vi "NXT_MIDBRAIN REVERSE.vi"(2 "_sensorData":T2={"_irData"={"_irDistance"=0, "_irHeading"=0, "_irTimestamp"=0}, "_batteryVoltage"=0, "_NXTButtonStates"=[FALSE, FALSE, FALSE]}, 3 "Behavior #":i32, 4 "Previous Motor Position":T1={"_rudderCommand"=7, "_propCommand"=7, "_irServoCommand"=7}, 5 "Behavior Weights":T4=[0, 0, 0, 0, 0, 0]) -> (0 "Rudder Command":i32, 1 "Behavior Output":T5)   [LabVIEW 2012]
uses:
  behaviorOutput_t.ctl
  behaviorWeights_t.ctl
  sensorData_t.ctl
  irData_t.ctl
  motorCommands_t.ctl
panel:
  in  "greater250":i32
  in  "Goodness":i32=50
  in  "lessthat100":i32
  in  "between150_100":i32
  in  "between200_150":i32
  in  "between250_200":i32
  in  "Speed":i32=1
  # "DEBUG"
  # "L\nE\nF\nT"
  # "C\nE\nN\nT\nE\nR"
  # "R\nI\nG\nH\nT"
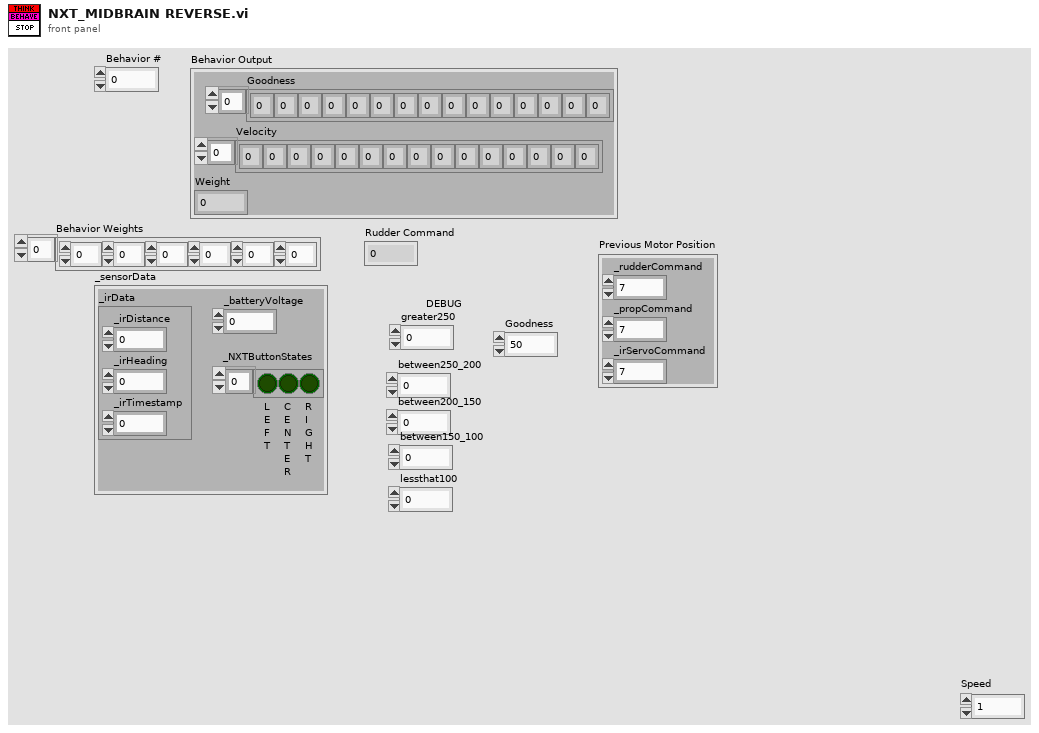
[diagram p1: front panel]
types:
  T1 = typedef "motorCommands_t.ctl" = cluster{"_rudderCommand":i8, "_propCommand":i8, "_irServoCommand":i8}
  T2 = typedef "sensorData_t.ctl" = cluster{"_irData":T3, "_batteryVoltage":i32, "_NXTButtonStates":bool[]}
  T3 = typedef "irData_t.ctl" = cluster{"_irDistance":i32, "_irHeading":i32, "_irTimestamp":u32}
  T4 = typedef "behaviorWeights_t.ctl" = i8[]
  T5 = typedef "behaviorOutput_t.ctl" = cluster{"Goodness":i8[], "Velocity":i8[], "Weight":i8}
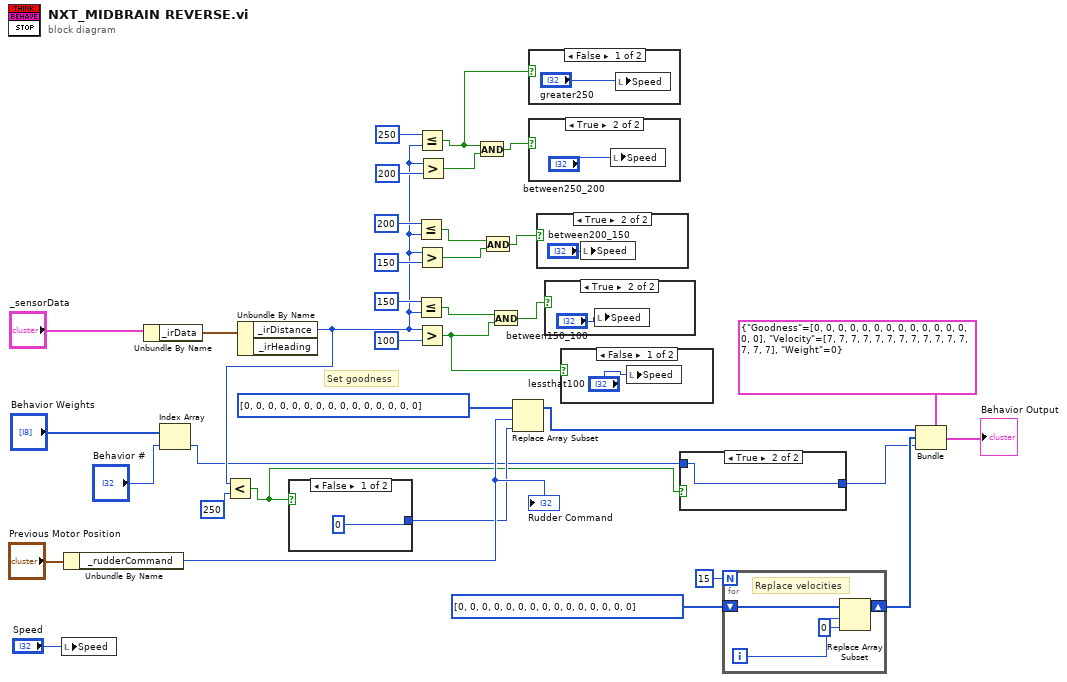
[diagram p0: block diagram]
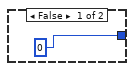
[diagram p2: hidden frame]
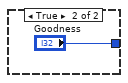
[diagram p3: hidden frame]
diagram:
  # "Set goodness"
  n1 = local write "Speed"("Speed") -> ()
  n2 = Unbundle By Name("Previous Motor Position") -> ("_rudderCommand"=w10:i8)
  "Rudder Command" <- w10
  n3 = Unbundle By Name("_sensorData") -> ("_irData"=w30:T3)
  n4 = Index Array(array="Behavior Weights", index="Behavior #") -> (element=w2:i8)
  n5 = Unbundle By Name(w30) -> ("_irDistance"=w4:i32)  [unwired: 1 out]
  n6 = Less?(x=w4, y=250) -> (x < y?=w3:bool)
  n7 = case shown="False" w3 {
    tunnel: [0 ("Numeric 2") "Goodness"] -> w8
    frame False {
    }
    frame True {
    }
  }
  n8 = Less Or Equal?(x=200 ("y"), y=w4) -> (x <= y?=w18:bool)
  n9 = Less Or Equal?(x=150 ("y"), y=w4) -> (x <= y?=w16:bool)
  n10 = Less Or Equal?(x=250 ("y"), y=w4) -> (x <= y?=w14:bool)
  n11 = Greater?(x=w4, y=150) -> (0:w17:bool)
  n12 = Greater?(x=w4, y=100) -> (0:w9:bool)
  n13 = Greater?(x=w4, y=200) -> (0:w19:bool)
  n14 = And(x=w14, y=w19) -> (x .and. y?=w15:bool)
  n15 = And(x=w18, y=w17) -> (x .and. y?=w13:bool)
  n16 = And(x=w16, y=w9) -> (x .and. y?=w12:bool)
  n17 = Replace Array Subset(array=i8[] [0, 0, 0, 0, 0, 0, 0, 0, 0, 0, 0, 0, 0, 0, 0] ("Goodness"), new element=w8, index=w10) -> (w27:i8[])
  n18 = case shown="False" w14 {
    frame False {
      n19 = local write "Speed"("greater250") -> ()
    }
    frame True {
    }
  }
  n20 = case shown="True" w15 {
    frame False {
    }
    frame True {
      n21 = local write "Speed"("between250_200") -> ()
    }
  }
  n22 = case shown="True" w13 {
    frame False {
    }
    frame True {
      n23 = local write "Speed"("between200_150") -> ()
    }
  }
  n24 = case shown="True" w12 {
    frame False {
    }
    frame True {
      n25 = local write "Speed"("between150_100") -> ()
    }
  }
  n26 = case shown="False" w9 {
    frame False {
      n27 = local write "Speed"("lessthat100") -> ()
    }
    frame True {
    }
  }
  n28 = case shown="True" w3 {
    tunnel: w2 -> [_ w44]
    tunnel: [0 w44] -> w1
    frame False {
    }
    frame True {
    }
  }
  n29 = for {
    N: 15 -> [_]
    shift-right: [w48] -> w26
    shift-left: i8[] [0, 0, 0, 0, 0, 0, 0, 0, 0, 0, 0, 0, 0, 0, 0] ("Goodness") -> [w46]
    i -> [w45]
    # "Replace velocities"
    n30 = Replace Array Subset(array=w46, new element=i8 0 ("new element/subarray"), index=w45) -> (w48:i8[])
  }
  n31 = Bundle(cluster=T5 {"Goodness"=[0, 0, 0, 0, 0, 0, 0, 0, 0, 0, 0, 0, 0, 0, 0], "Velocity"=[7, 7, 7, 7, 7, 7, 7, 7, 7, 7, 7, 7, 7, 7, 7], "Weight"=0} ("Behavior Output"), "Goodness"=w27, "Velocity"=w26, "Weight"=w1) -> (→"Behavior Output":T5)
